vi "Vortex.vi"(11 "General settings":T1) -> (2 "Vortex":dbl[][](array[numeric]))   [LabVIEW 2018]
uses:
  Controls/General Setting.ctl
  Controls/Buttons/Running Button.ctl
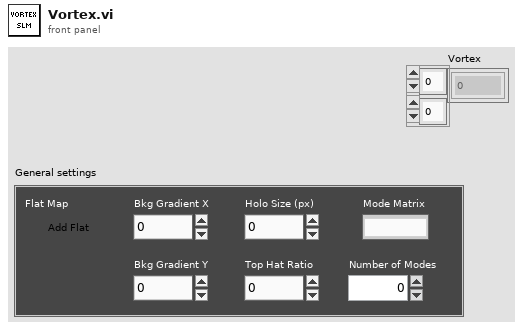
[diagram p1: front panel]
types:
  T1 = typedef "General Setting.ctl" = cluster{"Flat Map":T2, "Bkg Gradient X":dbl, "Bkg Gradient Y":dbl, "Holo Size (px)":i32, "Top Hat Ratio":dbl, "Number of Modes":i8, "Mode Matrix":u16}
  T2 = typedef "Running Button.ctl" = bool
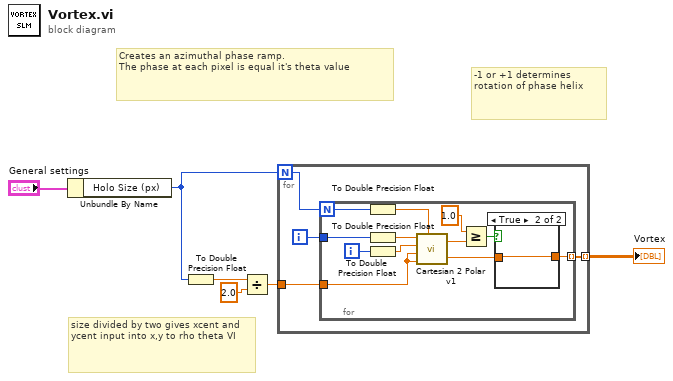
[diagram p0: block diagram]
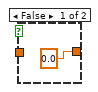
[diagram p2: hidden frame]
diagram:
  # "-1 or +1 determines \nrotation of phase helix"
  # "Creates an azimuthal phase ramp.\nThe phase at each pixel is equal it's theta value"
  # "size divided by two gives xcent and ycent input into x,y to rho theta VI"
  n1 = Unbundle By Name("General settings") -> ("Holo Size (px)"=w3:i32)
  n2 = To Double Precision Float(number=w3) -> (double precision float=w2:dbl)
  n3 = Divide(x=w2, y=2.0) -> (x/y=w6:dbl)
  n4 = for {
    N: w3 -> [w7]
    tunnel: [w9] -> w1 mode=indexing
    tunnel: w6 -> [w8]
    i -> [w10]
    n5 = for {
      N: w7 -> [w15]
      tunnel: w10 -> [w21]
      tunnel: [w14] -> w9 mode=indexing
      tunnel: w8 -> [w16]
      i -> [w22]
      n6 = To Double Precision Float(number=w15) -> (double precision float=w13:dbl)
      n7 = To Double Precision Float(number=w21) -> (double precision float=w12:dbl)
      n8 = To Double Precision Float(number=w22) -> (double precision float=w11:dbl)
      n9 = call "Cartesian 2 Polar v1.vi"("x"=w12, "y"=w11, "xcent"=w16, "ycent"=w16, "diam"=w13) -> ("rho"=w18:dbl, "theta"=w20:dbl)
      n10 = Greater Or Equal?(x=1.0, y=w18) -> (x >= y?=w19:bool)
      n11 = case shown="True" w19 {
        tunnel: w20 -> [_ w24]
        tunnel: [0.0 ("zernike") w24] -> w14
        frame False {
        }
        frame True {
        }
      }
    }
  }
  "Vortex" <- w1
